vi "HXG_radial profile_new.vi"(11 "QI 传递变量输入":T1) -> (1 "radial profile":dbl[](array[numeric]), 2 "array R":dbl[](array[numeric]), 3 "QI 传递变量输出":T1)   [LabVIEW 2017]
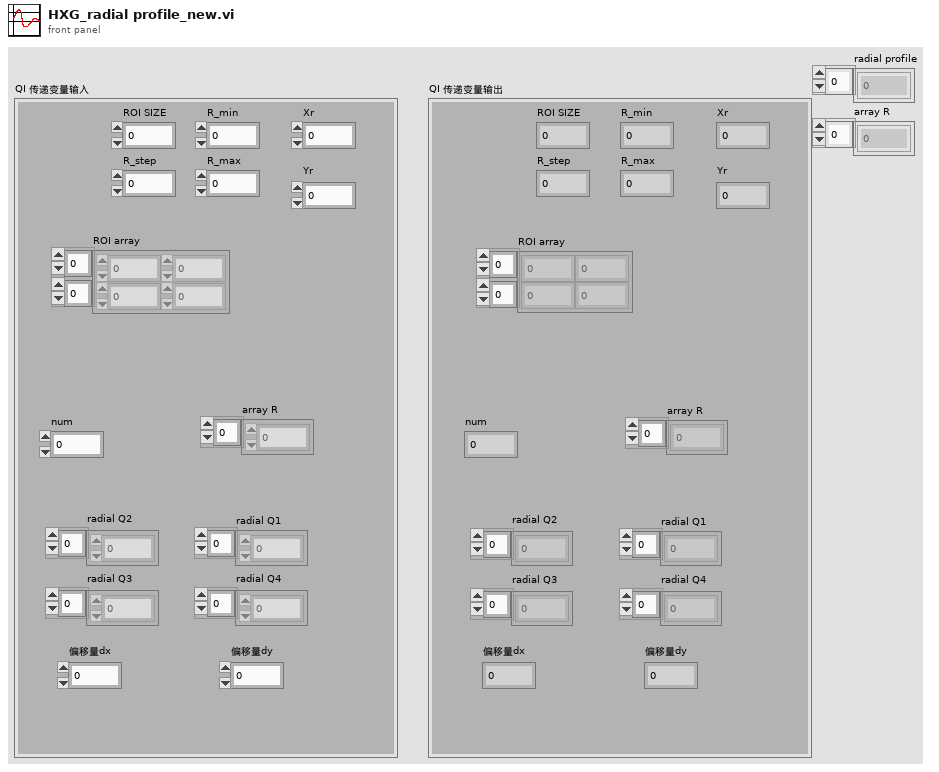
[diagram p1: front panel]
types:
  T1 = typedef "QI 传递变量.ctl" = cluster{"ROI SIZE":i32, "R_step":dbl, "R_min":dbl, "R_max":dbl, "num":dbl, "array R":dbl[], "radial Q1":dbl[], "radial Q2":dbl[], "radial Q3":dbl[], "radial Q4":dbl[], "偏移量dx":dbl, "偏移量dy":dbl, "ROI array":sgl[][], "Xr":dbl, "Yr":dbl}
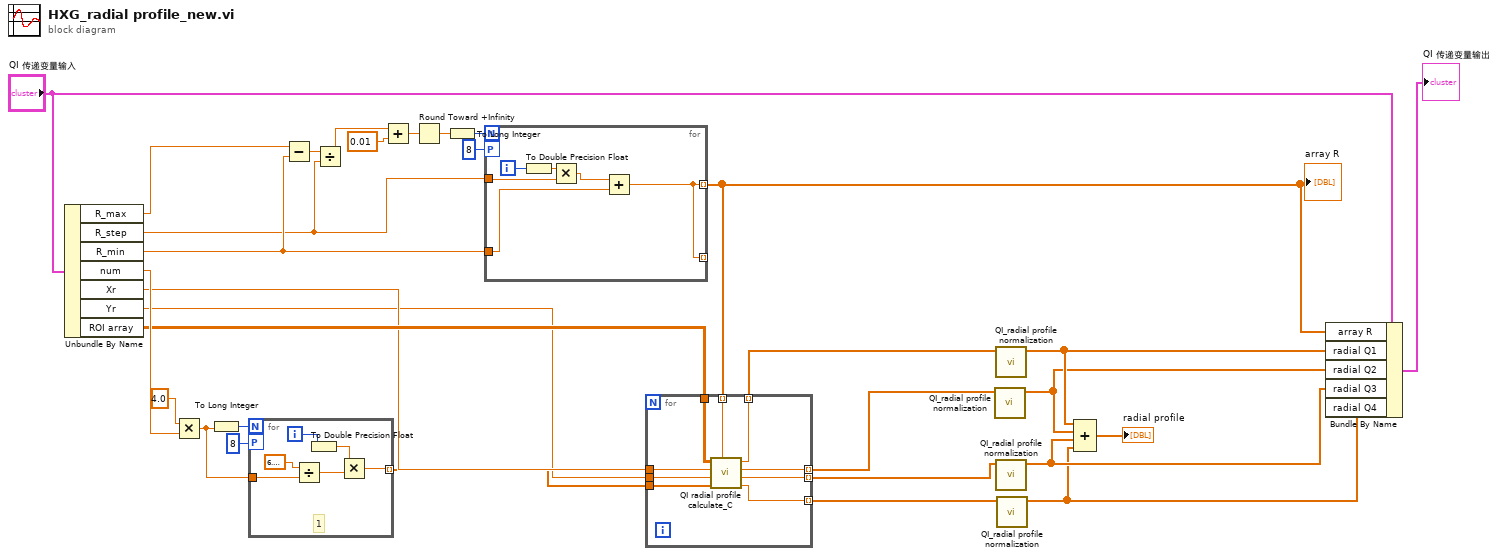
[diagram p0: block diagram]
diagram:
  n1 = Unbundle By Name("QI 传递变量输入") -> ("R_max"=w29:dbl, "R_step"=w26:dbl, "R_min"=w28:dbl, "num"=w13:dbl, "Xr"=w7:dbl, "Yr"=w6:dbl, "ROI array"=w8:sgl[][])
  n2 = Multiply(x=4.0, y=w13) -> (x*y=w14:dbl)
  n3 = To Long Integer(number=w14) -> (32bit integer=w16:i32)
  n4 = for {
    N: w16 -> [_]
    tunnel: w14 -> [w37]
    tunnel: [w33] -> w5 mode=indexing
    workers-P: 8 -> [_]
    i -> [w35]
    # "1"
    n5 = Divide(x=6.283185307179586, y=w37) -> (x/y=w36:dbl)
    n6 = To Double Precision Float(number=w35) -> (double precision float=w34:dbl)
    n7 = Multiply(x=w34, y=w36) -> (x*y=w33:dbl)
  }
  n8 = Subtract(x=w29, y=w28) -> (x-y=w27:dbl)
  n9 = Divide(x=w27, y=w26) -> (x/y=w25:dbl)
  n10 = Add(x=w25, y=0.01) -> (x+y=w23:dbl)
  n11 = Round Toward +Infinity(x=w23) -> (ceil(x): smallest int >= x=w22:dbl)
  n12 = To Long Integer(number=w22) -> (32bit integer=w21:i32)
  n13 = for "For循环" {
    N: w21 -> [_]
    tunnel: w28 -> [w40]
    tunnel: w26 -> [w42]
    tunnel: [w38] -> w9 mode=indexing
    tunnel: [w38] -> _ mode=indexing
    workers-P: 8 -> [_]
    i -> [w43]
    n14 = To Double Precision Float(number=w43) -> (double precision float=w39:dbl)
    n15 = Multiply(x=w39, y=w42) -> (x*y=w41:dbl)
    n16 = Add(x=w41, y=w40) -> (x+y=w38:dbl)
  }
  "array R" <- w9
  n17 = for {
    tunnel: w9 -> [w52] mode=indexing
    tunnel: w8 -> [w51]
    tunnel: w7 -> [w50]
    tunnel: w6 -> [w49]
    tunnel: w5 -> [w48]
    tunnel: [w47] -> w4 mode=indexing
    tunnel: [w46] -> w3 mode=indexing
    tunnel: [w45] -> w2 mode=indexing
    tunnel: [w44] -> w1 mode=indexing
    n18 = call "QI radial profile calculate_C.vi"("r"=w52, "rad"=w48, "Yr"=w49, "Xr"=w50, "ROI array"=w51) -> ("mean4"=w44:dbl, "mean3"=w45:dbl, "mean2"=w46:dbl, "mean1"=w47:dbl)  [unwired: 3 in]
  }
  n19 = call "QI_radial profile normalization.vi"("rp输入"=w3) -> ("rp输出"=w19:dbl[])  [unwired: 10 in]
  n20 = call "QI_radial profile normalization.vi"("rp输入"=w4) -> ("rp输出"=w20:dbl[])  [unwired: 10 in]
  n21 = call "QI_radial profile normalization.vi"("rp输入"=w2) -> ("rp输出"=w18:dbl[])  [unwired: 10 in]
  n22 = call "QI_radial profile normalization.vi"("rp输入"=w1) -> ("rp输出"=w17:dbl[])  [unwired: 10 in]
  n23 = Compound Arithmetic op=ADD(w20, w19, w18, w17) -> (→"radial profile":dbl[])
  n24 = Bundle By Name(cluster="QI 传递变量输入", "array R"=w9, "radial Q1"=w20, "radial Q2"=w19, "radial Q3"=w18, "radial Q4"=w17) -> (→"QI 传递变量输出":T1)
